vi "SaveConfig.vi"(8 "error in (no error)":errorcluster, 11 "GRMActor in":refnum<class "CameraController.lvclass">) -> (0 "error out":errorcluster, 3 "GRMActor out":refnum<class "CameraController.lvclass">)   [LabVIEW 2020, in "CameraController.lvlib" / "CameraController.lvclass"]
uses:
  CameraController.lvclass
  Model/Hardware Abstraction Layer/Component/GenericActor/GenericActor/GenericController.lvclass
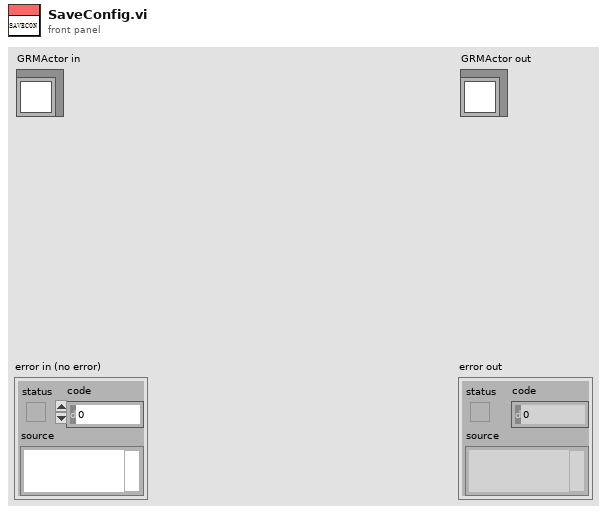
[diagram p1: front panel]
types:
  T1 = typedef "NI_LVConfig.lvlib/Config Data RefNum.ctl" = refnum<k1>
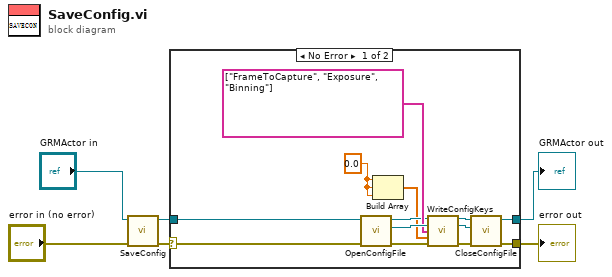
[diagram p0: block diagram]
diagram:
  n1 = call-parent "SaveConfig.vi"("error in (no error)"="error in (no error)", "GRMActor in"="GRMActor in") -> ("error out"=w3:errorcluster, "GRMActor out"=w4:refnum<class "CameraController.lvclass">)  [unwired: 8 in]
  n2 = case shown="No Error" w3 {
    selector: w3 -> [w10 w20]
    tunnel: [w17 w20] -> w1
    tunnel: [w15 w21] -> w2
    tunnel: w4 -> [w8 w21]
    frame No Error {
      w7 = 0.0 ("element")
      n3 = call-dynamic "OpenConfigFile.vi"("error in (no error)"=w10, "GRMActor in"=w8) -> ("error out"=w18:errorcluster, "refnum"=w14:T1, "GRMActor out"=w11:refnum<class "CameraController.lvclass">)  [unwired: 7 in]
      n4 = Build Array(w7, w7, w7) -> (w9:dbl[])
      n5 = call-dynamic "WriteConfigKeys.vi"("GRMActor in"=w11, "Config Refnum"=w14, "Keys"=string[] ["FrameToCapture", "Exposure", "Binning"] ("Values"), "IntValue"=w9, "error in (no error)"=w18) -> ("GRMActor out"=w16:refnum<class "CameraController.lvclass">, "Config Refnum dup"=w13:T1, "error out"=w19:errorcluster)  [unwired: 8 in]
      n6 = call-dynamic "CloseConfigFile.vi"("error in (no error)"=w19, "refnum"=w13, "GRMActor in"=w16) -> ("error out"=w17:errorcluster, "GRMActor out"=w15:refnum<class "CameraController.lvclass">)  [unwired: 7 in]
    }
    frame Error {
    }
  }
  "error out" <- w1
  "GRMActor out" <- w2
